vi "FrontEnd_Module.vi"() -> ()   [LabVIEW 2023]
uses:
  Controls/Queue_Operation_Select.ctl
  Controls/Quantity_Data.ctl
  Controls/State_and_Data.ctl
  Controls/Select_Preference.ctl
  <vilib>/Utility/file.llb/Read Delimited Spreadsheet (string).vi
  Controls/Coffee_Machine_Data.ctl
panel:
  out "Error_Out":errorcluster
  in  "Error_In":errorcluster
  in  "Power":bool
  out "Dispaly":T1 {"Dispenser" scale=0.0..80.0; "Chamber" scale=0.0..80.0}
  in  "Selector":T2 {"Select_Bevarage" scale=0.0..2.0}
  # "Coffee"
  # "Latte"
  # "Hot Water"
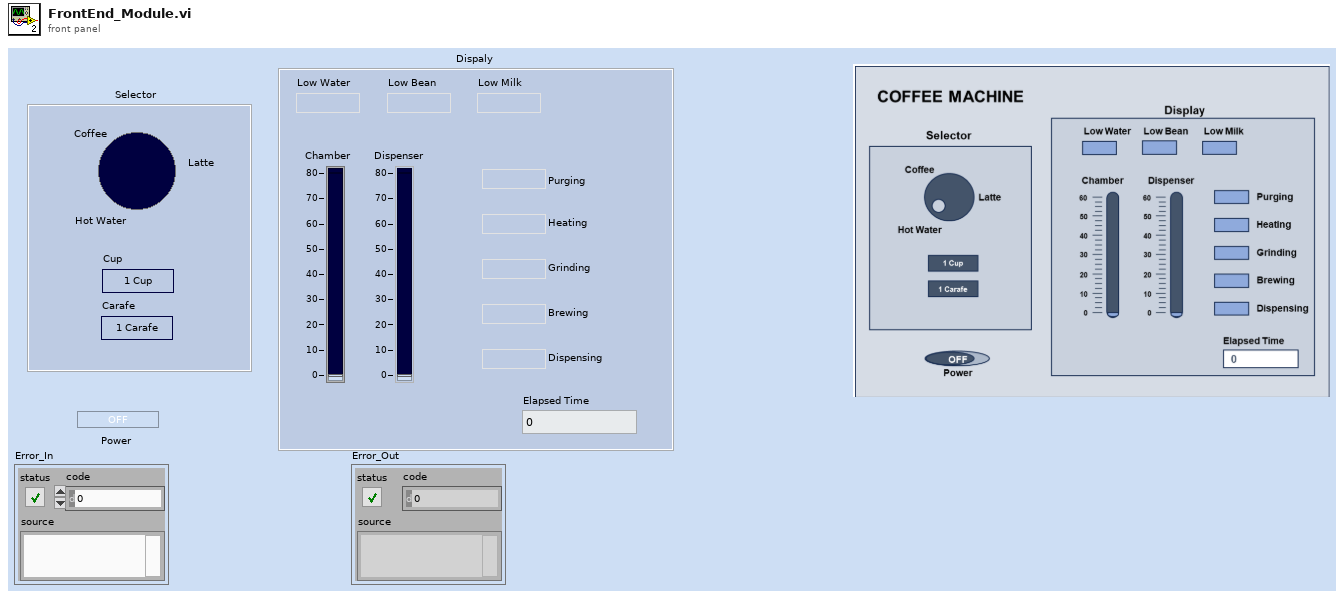
[diagram p1: front panel]
types:
  T1 = cluster{"Low_Water":bool, "Low_Bean":bool, "Low_Milk":bool, "Chamber":dbl, "Dispenser":dbl, "Purging":bool, "Heating":bool, "Grinding":bool, "Brewing":bool, "Dispensing":bool, "Elapsed_Time":dbl}
  T2 = typedef "Select_Preference.ctl" = cluster{"Select_Bevarage":i32, "Cup":bool, "Carafe":bool}
  T3 = typedef "Coffee_Machine_Data.ctl" = cluster{"Backend_Data":T4, "Selector":T2, "Cup_Unit":dbl, "Carafe_Unit":dbl, "Ingreedient_File_PAth":path, "Process_Needed":string[], "Indredient_Needed":string[], "Time_Needed":string[], "State_and_Data":T5}
  T4 = typedef "Quantity_Data.ctl" = cluster{"Level":cluster{"Water_Level":dbl, "Bean_Level":dbl, "Milk_Level":dbl}, "Total_Cups":dbl}
  T5 = typedef "State_and_Data.ctl" = cluster{"State":string, "Data":variant}
  T6 = typedef "Queue_Operation_Select.ctl" = enum16{"Obtain_Queue", "Enqueue", "Enqueue_First", "Enqueue_N", "Lossy_Enqueue", "Preview", "Queue_Status", "Dequeue", "Flush", "Release_Queue"}
  T7 = cluster{"Water_Level":dbl, "Bean_Level":dbl, "Milk_Level":dbl}
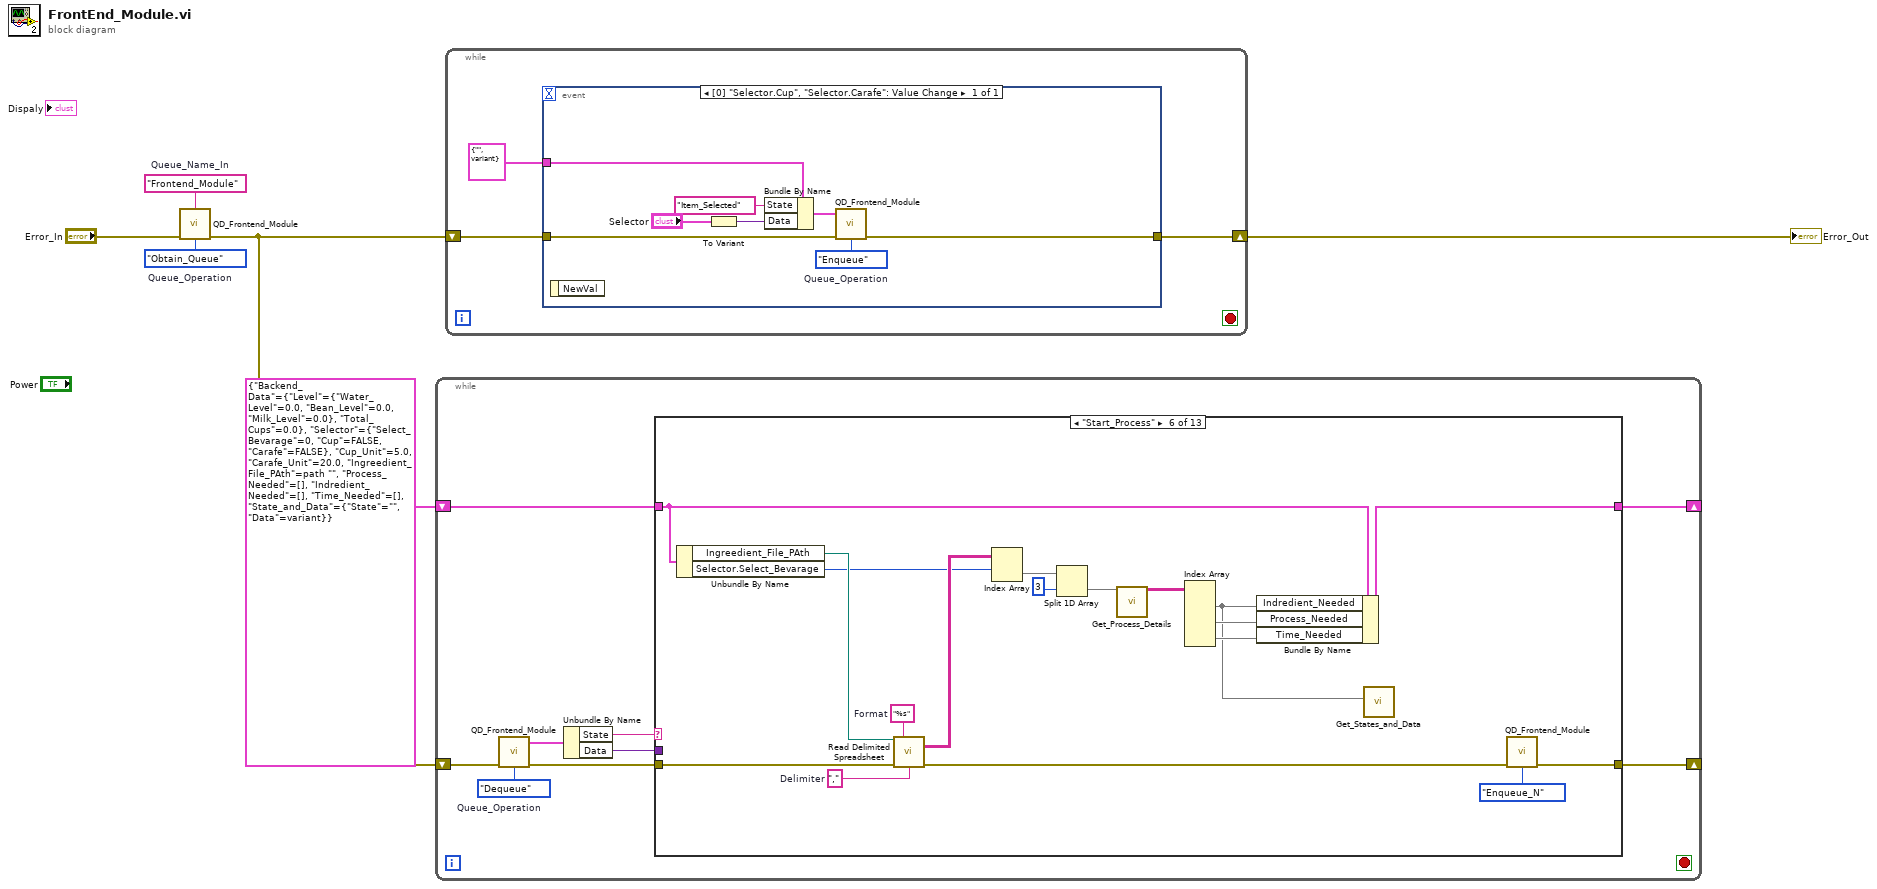
[diagram p0: block diagram]
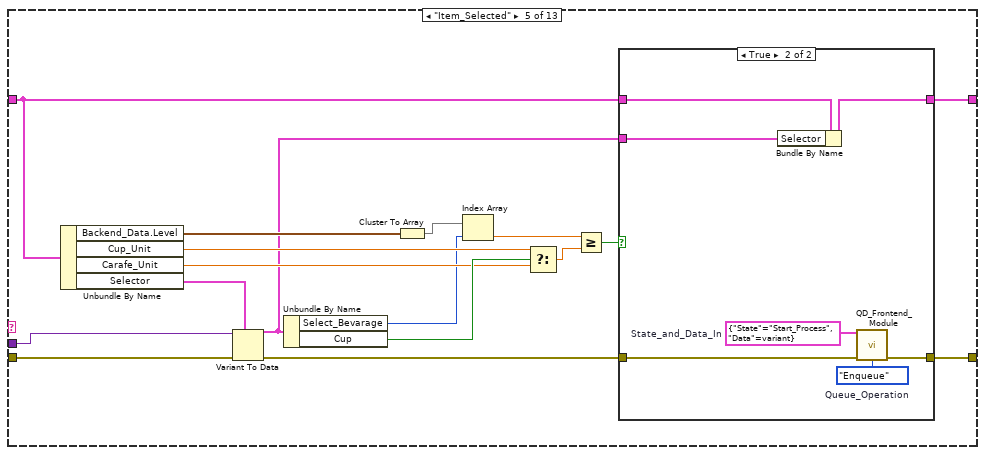
[diagram p6: hidden frame]
diagram:
  w4 = "Frontend_Module"  # Queue_Name_In
  w5 = Queue_Operation_Select."Obtain_Queue"  # Queue_Operation
  n1 = call "QD_Frontend_Module.vi"("Queue_Name_In"=w4, "Error_In"="Error_In", "Queue_Operation"=w5) -> ("Error_Out"=w2:errorcluster)  [unwired: 10 in, 2 out]
  n2 = while {
    shift-right: [w7] -> _
    shift-left: T3 {"Backend_Data"={"Level"={"Water_Level"=0.0, "Bean_Level"=0.0, "Milk_Level"=0.0}, "Total_Cups"=0.0}, "Selector"={"Select_Bevarage"=0, "Cup"=FALSE, "Carafe"=FALSE}, "Cup_Unit"=5.0, "Carafe_Unit"=20.0, "Ingreedient_File_PAth"=path "", "Process_Needed"=[], "Indredient_Needed"=[], "Time_Needed"=[], "State_and_Data"={"State"="", "Data"=variant}} -> [w8]
    shift-right: [w9] -> _
    shift-left: w2 -> [w15]
    stop <- _ stop-if-true
    w13 = Queue_Operation_Select."Dequeue"  # Queue_Operation
    n3 = call "QD_Frontend_Module.vi"("Error_In"=w15, "Queue_Operation"=w13) -> ("State_and_Data_Out"=w12:T5, "Error_Out"=w14:errorcluster)  [unwired: 11 in, 1 out]
    n4 = Unbundle By Name(w12) -> ("State"=w11:string, "Data"=w10:variant)
    n5 = case shown="\"Start_Process\"" w11 {
      tunnel: w14 -> [w17 w19 w21 w23 w40 w67 w69 w71 w73 w75 w77 w79 w81]
      tunnel: w10 -> [_ _ _ _ w39 _ _ _ _ _ _ _ _]
      tunnel: [w17 w19 w21 w23 w33 w53 w69 w71 w73 w75 w77 w79 w81] -> w9
      tunnel: w8 -> [w16 w18 w20 w22 w26 w50 w68 w70 w72 w74 w76 w78 w80]
      tunnel: [w16 w18 w20 w22 w27 w56 w68 w70 w72 w74 w76 w78 w80] -> w7
      frame "False", Default {
      }
      frame "Initialize" {
      }
      frame "Disable_and_Enable" {
      }
      frame "FP_Update" {
      }
      frame "Item_Selected" {
        n6 = Unbundle By Name(w26) -> ("Backend_Data.Level"=w31:T7, "Cup_Unit"=w37:dbl, "Carafe_Unit"=w36:dbl, "Selector"=w25:T2)
        n7 = Variant To Data(error in=w40, type=w25, Variant=w39) -> (data=w24:T2, error out=w32:errorcluster)
        n8 = Unbundle By Name(w24) -> ("Select_Bevarage"=w29:i32, "Cup"=w38:bool)
        n9 = Cluster To Array(cluster=w31) -> (array=w30:dbl[])
        n10 = Index Array(array=w30, index=w29) -> (element=w28:dbl)
        n11 = Select(t=w37, s=w38, f=w36) -> (s? t:f=w34:dbl)
        n12 = Greater Or Equal?(x=w28, y=w34) -> (x >= y?=w35:bool)
        n13 = case shown="True" w35 {
          tunnel: [w41 w45] -> w33
          tunnel: w32 -> [w41 w49]
          tunnel: [w42 w47] -> w27
          tunnel: w26 -> [w42 w48]
          tunnel: w24 -> [_ w46]
          frame False {
          }
          frame True {
            w43 = T5 {"State"="Start_Process", "Data"=variant}  # State_and_Data_In
            w44 = Queue_Operation_Select."Enqueue"  # Queue_Operation
            n14 = Bundle By Name(cluster=w48, "Selector"=w46) -> (w47:T3)
            n15 = call "QD_Frontend_Module.vi"("State_and_Data_In"=w43, "Error_In"=w49, "Queue_Operation"=w44) -> ("Error_Out"=w45:errorcluster)  [unwired: 10 in, 2 out]
          }
        }
      }
      frame "Start_Process" {
        w63 = "%s"  # Format
        w64 = ","  # Delimiter
        n16 = Unbundle By Name(w50) -> ("Ingreedient_File_PAth"=w65:path, "Selector.Select_Bevarage"=w61:i32)
        n17 = call-poly <vilib>:"Read Delimited Spreadsheet.vi"("file path (dialog if empty)"=w65, "format (%s)"=w63, "error in (no error)"=w67, "delimiter (\\t)"=w64) -> ("all rows"=w62:string[][], "error out"=w66:errorcluster)  [unwired: 6 in, 4 out]
        n18 = Index Array(array=w62, index (row)=w61) -> (element=w60:string[])  [unwired: 1 in]
        n19 = Split 1D Array(array=w60, index=3) -> (second subarray=w58:string[])  [unwired: 1 out]
        n20 = call "Get_Process_Details.vi"("Process_Data"=w58) -> ("Needs"=w57:string[][])  [unwired: 14 in]
        n21 = Index Array(array=w57) -> (element #1=w51:string[], element #2=w55:string[], element #3=w54:string[])  [unwired: 6 in]
        n22 = Bundle By Name(cluster=w50, "Indredient_Needed"=w51, "Process_Needed"=w55, "Time_Needed"=w54) -> (w56:T3)
        n23 = call "Get_States_and_Data.vi"("Ingredient_Needed"=w51) -> ()  [unwired: 11 in]
        n24 = call "QD_Frontend_Module.vi"("Error_In"=w66, "Queue_Operation"=Queue_Operation_Select."Enqueue_N") -> ("Error_Out"=w53:errorcluster)  [unwired: 11 in, 2 out]
      }
      frame "Water" {
      }
      frame "Bean" {
      }
      frame "Milk" {
      }
      frame "Preparing" {
      }
      frame "Error" {
      }
      frame "Request_Exit" {
      }
      frame "Exit" {
      }
    }
  }
  n25 = while {
    shift-right: [w84] -> w3
    shift-left: w2 -> [w83]
    stop <- _ stop-if-true
    n26 = event shown="[0] \"Selector.Cup\", \"Selector.Carafe\": Value Change" {
      selector: _ -> [_]
      dyn-events: _ -> [_]
      timeout: _ -> [_]
      tunnel: [w91] -> w84
      tunnel: w83 -> [w92]
      tunnel: T5 {"State"="", "Data"=variant} ("State_and_Data") -> [w86]
      event Value Change {
        w90 = Queue_Operation_Select."Enqueue"  # Queue_Operation
        n27 = event-data() -> ()  [unwired: 1 in, 1 out]
        n28 = To Variant(anything="Selector") -> (Variant=w88:variant)
        n29 = Bundle By Name(cluster=w86, "State"="Item_Selected", "Data"=w88) -> (w87:T5)
        n30 = call "QD_Frontend_Module.vi"("State_and_Data_In"=w87, "Error_In"=w92, "Queue_Operation"=w90) -> ("Error_Out"=w91:errorcluster)  [unwired: 10 in, 2 out]
      }
    }
  }
  "Error_Out" <- w3
